vi "Test Servo 1.vi"() -> ()   [LabVIEW 2014]
uses:
  LabVIEW-Universal-Transcriptor-ServoLibrary/ServoDatatype.lvclass
panel:
  out "Error Out":errorcluster
  in  "Error In":errorcluster
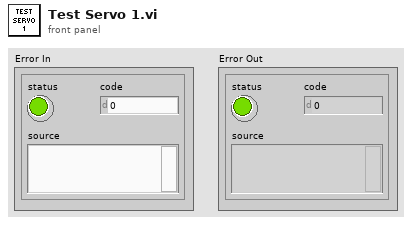
[diagram p1: front panel]
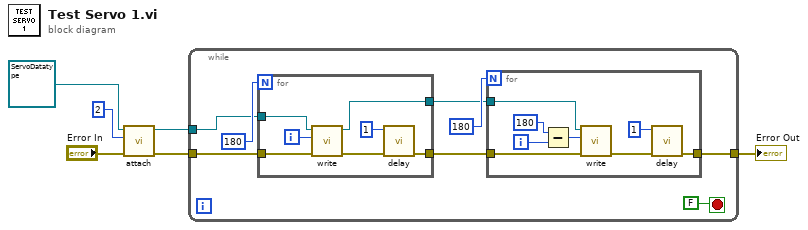
[diagram p0: block diagram]
diagram:
  n1 = call-dynamic "attach.vi"("error in (no error)"="Error In", "pin number"=2, "Servo in"=refnum<class "ServoDatatype.lvclass"> refnum) -> ("error out"=w3:errorcluster, "Servo out"=w2:refnum<class "ServoDatatype.lvclass">)  [unwired: 6 in, 1 out]
  n2 = while {
    tunnel: w3 -> [w12]
    tunnel: w2 -> [w13]
    tunnel: [w7] -> w1
    stop <- FALSE stop-if-true
    n3 = for {
      N: 180 -> [_]
      tunnel: w13 -> [w29]
      tunnel: w12 -> [w27]
      tunnel: [w26] -> w10
      tunnel: [w23] -> w8
      i -> [w28]
      n4 = call-dynamic "write.vi"("error in (no error)"=w27, "value"=w28, "ServoDatatype in"=w29) -> ("error out"=w24:errorcluster, "ServoDatatype out"=w26:refnum<class "ServoDatatype.lvclass">)  [unwired: 7 in]
      n5 = call <vilib>:"delay.vi"("Error In"=w24, "time (ms)"=1) -> ("Error Out"=w23:errorcluster)  [unwired: 9 in]
    }
    n6 = for {
      N: 180 -> [_]
      tunnel: w10 -> [w22]
      tunnel: w8 -> [w21]
      tunnel: [w15] -> w7
      i -> [w19]
      n7 = Subtract(x=180, y=w19) -> (x-y=w18:i32)
      n8 = call-dynamic "write.vi"("error in (no error)"=w21, "value"=w18, "ServoDatatype in"=w22) -> ("error out"=w16:errorcluster)  [unwired: 7 in, 1 out]
      n9 = call <vilib>:"delay.vi"("Error In"=w16, "time (ms)"=1) -> ("Error Out"=w15:errorcluster)  [unwired: 9 in]
    }
  }
  "Error Out" <- w1
